vi "rg_for_command_mem.vi"(0 "WR":bool, 1 "RD":bool, 2 "input":T1, 3 "такты":bool, 4 "R":bool) -> (5 "output":T2)   [LabVIEW 2013]
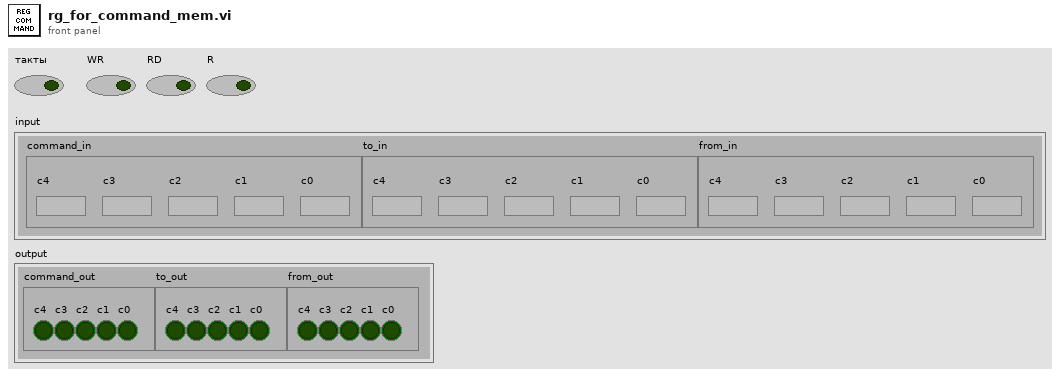
[diagram p1: front panel]
types:
  T1 = cluster{"command_in":cluster{"c4":bool, "c3":bool, "c2":bool, "c1":bool, "c0":bool}, "to_in":cluster{"c4":bool, "c3":bool, "c2":bool, "c1":bool, "c0":bool}, "from_in":cluster{"c4":bool, "c3":bool, "c2":bool, "c1":bool, "c0":bool}}
  T2 = cluster{"command_out":cluster{"c4":bool, "c3":bool, "c2":bool, "c1":bool, "c0":bool}, "to_out":cluster{"c4":bool, "c3":bool, "c2":bool, "c1":bool, "c0":bool}, "from_out":cluster{"c4":bool, "c3":bool, "c2":bool, "c1":bool, "c0":bool}}
  T3 = cluster{"c4":bool, "c3":bool, "c2":bool, "c1":bool, "c0":bool}
  T4 = cluster{"Q":bool, "Q":bool, "Q":bool, "Q":bool, "Q":bool}
  T5 = cluster{cluster{"Q":bool, "Q":bool, "Q":bool, "Q":bool, "Q":bool}, cluster{"Q":bool, "Q":bool, "Q":bool, "Q":bool, "Q":bool}, cluster{"Q":bool, "Q":bool, "Q":bool, "Q":bool, "Q":bool}}
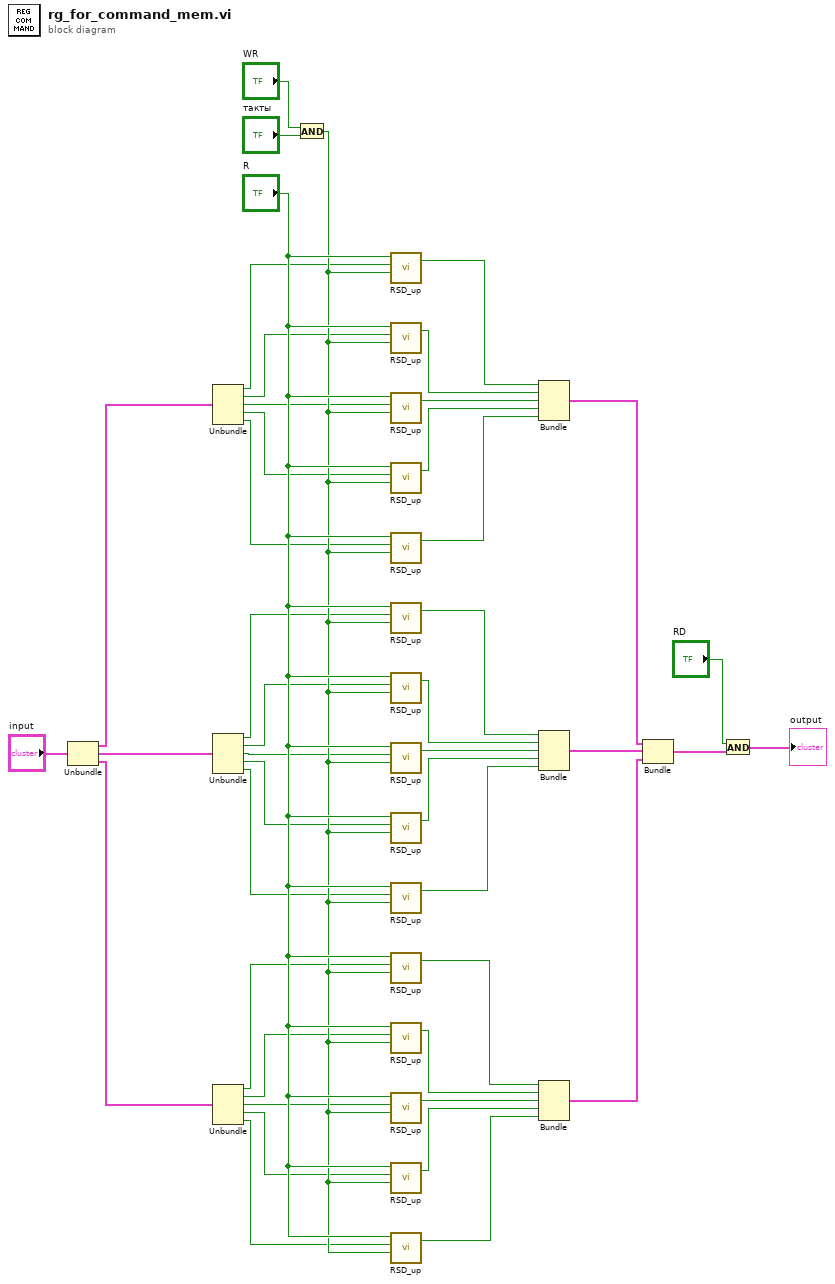
[diagram p0: block diagram]
diagram:
  n1 = Unbundle("input") -> ("command_in"=w2:T3, "to_in"=w3:T3, "from_in"=w1:T3)
  n2 = Unbundle(w2) -> ("c4"=w17:bool, "c3"=w16:bool, "c2"=w18:bool, "c1"=w14:bool, "c0"=w15:bool)
  n3 = Unbundle(w3) -> ("c4"=w12:bool, "c3"=w10:bool, "c2"=w13:bool, "c1"=w9:bool, "c0"=w11:bool)
  n4 = Unbundle(w1) -> ("c4"=w7:bool, "c3"=w5:bool, "c2"=w8:bool, "c1"=w4:bool, "c0"=w6:bool)
  n5 = And(x="WR", y="такты") -> (x .and. y?=w40:bool)
  n6 = call "RSD_up.vi"("C"=w40, "D"=w17, "R"="R") -> ("Q"=w38:bool)  [unwired: 1 in, 1 out]
  n7 = call "RSD_up.vi"("C"=w40, "D"=w16, "R"="R") -> ("Q"=w37:bool)  [unwired: 1 in, 1 out]
  n8 = call "RSD_up.vi"("C"=w40, "D"=w18, "R"="R") -> ("Q"=w39:bool)  [unwired: 1 in, 1 out]
  n9 = call "RSD_up.vi"("C"=w40, "D"=w14, "R"="R") -> ("Q"=w36:bool)  [unwired: 1 in, 1 out]
  n10 = call "RSD_up.vi"("C"=w40, "D"=w15, "R"="R") -> ("Q"=w35:bool)  [unwired: 1 in, 1 out]
  n11 = call "RSD_up.vi"("C"=w40, "D"=w12, "R"="R") -> ("Q"=w32:bool)  [unwired: 1 in, 1 out]
  n12 = call "RSD_up.vi"("C"=w40, "D"=w10, "R"="R") -> ("Q"=w33:bool)  [unwired: 1 in, 1 out]
  n13 = call "RSD_up.vi"("C"=w40, "D"=w13, "R"="R") -> ("Q"=w34:bool)  [unwired: 1 in, 1 out]
  n14 = call "RSD_up.vi"("C"=w40, "D"=w9, "R"="R") -> ("Q"=w30:bool)  [unwired: 1 in, 1 out]
  n15 = call "RSD_up.vi"("C"=w40, "D"=w11, "R"="R") -> ("Q"=w31:bool)  [unwired: 1 in, 1 out]
  n16 = call "RSD_up.vi"("C"=w40, "D"=w7, "R"="R") -> ("Q"=w26:bool)  [unwired: 1 in, 1 out]
  n17 = call "RSD_up.vi"("C"=w40, "D"=w5, "R"="R") -> ("Q"=w28:bool)  [unwired: 1 in, 1 out]
  n18 = call "RSD_up.vi"("C"=w40, "D"=w8, "R"="R") -> ("Q"=w29:bool)  [unwired: 1 in, 1 out]
  n19 = call "RSD_up.vi"("C"=w40, "D"=w4, "R"="R") -> ("Q"=w27:bool)  [unwired: 1 in, 1 out]
  n20 = call "RSD_up.vi"("C"=w40, "D"=w6, "R"="R") -> ("Q"=w25:bool)  [unwired: 1 in, 1 out]
  n21 = Bundle("Q"=w38, "Q"=w37, "Q"=w39, "Q"=w36, "Q"=w35) -> (w23:T4)  [unwired: 1 in]
  n22 = Bundle("Q"=w32, "Q"=w33, "Q"=w34, "Q"=w30, "Q"=w31) -> (w24:T4)  [unwired: 1 in]
  n23 = Bundle("Q"=w26, "Q"=w28, "Q"=w29, "Q"=w27, "Q"=w25) -> (w22:T4)  [unwired: 1 in]
  n24 = Bundle(w23, w24, w22) -> (w21:T5)  [unwired: 1 in]
  n25 = And(x="RD", y=w21) -> (x .and. y?=→"output":T5)
